vi "Tosca-2P-Frame Rate Counter.vi"(0 "TwoP":T1, 7 "2P Control":refnum<notifier>) -> (15 "error out":errorcluster)   [LabVIEW 2020]
uses:
  Tosca-2P Config.ctl
  <vilib>/DAQmx/read.llb/DAQmx Read (Counter 1D DBL 1Chan NSamp).vi
  <vilib>/Analysis/baseanly.llb/Mean (DBL).vi
  <vilib>/DAQmx/create/channels.llb/DAQmx Create Channel (CI-Period).vi
  <vilib>/DAQmx/configure/timing.llb/DAQmx Timing (Implicit).vi
  <vilib>/DAQmx/miscellaneous.llb/DAQmx Fill In Error Info.vi
  Tosca-2P-Globals.vi
  <vilib>/Analysis/NI_AALBase.lvlib
  <resource>/objmgr/daqmx.rc
panel:
  out "Frame rate (Hz)":dbl
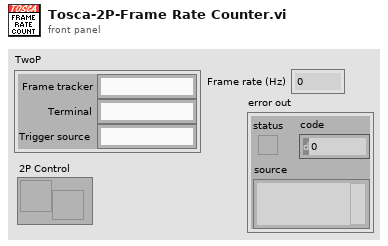
[diagram p1: front panel]
types:
  T1 = typedef "Tosca-2P Config.ctl" = cluster{"Frame tracker":string, "Terminal":string, "Trigger source":string}
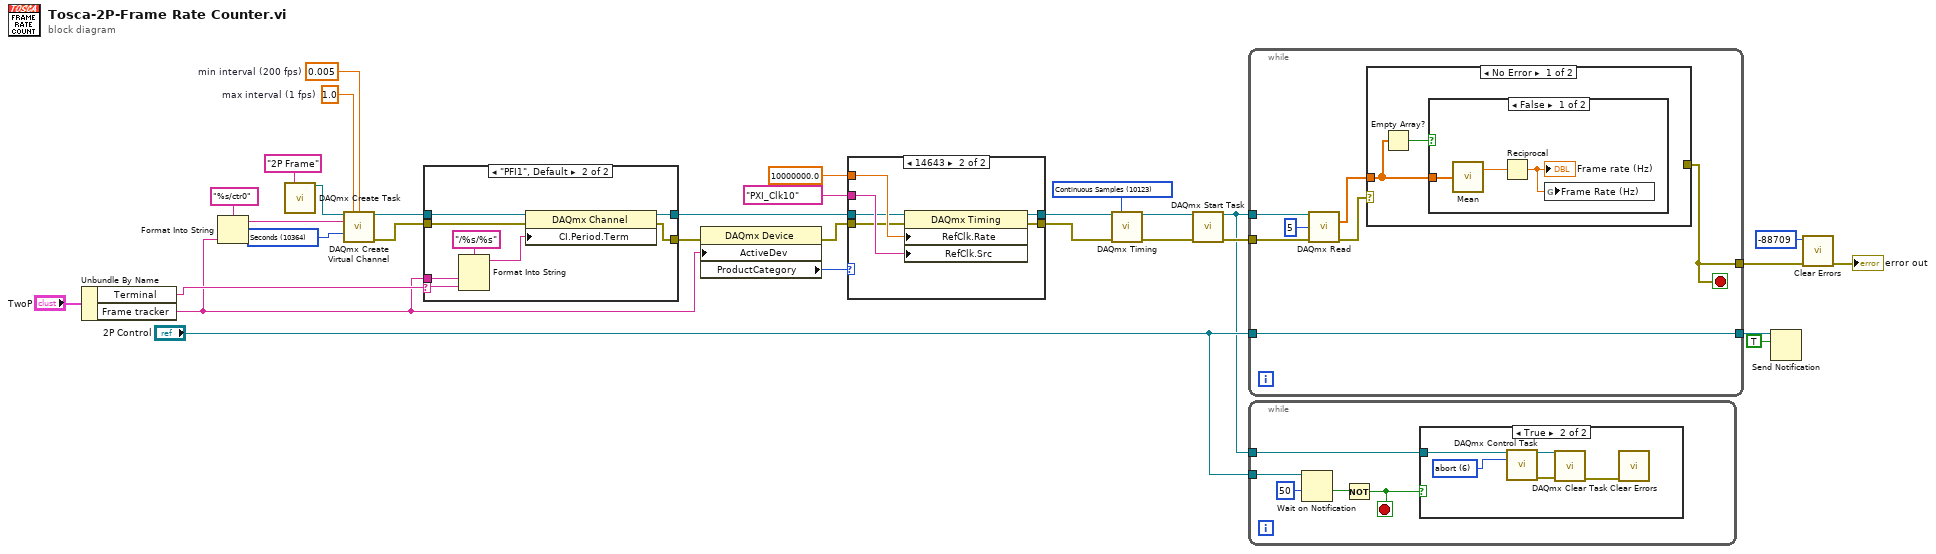
[diagram p0: block diagram]
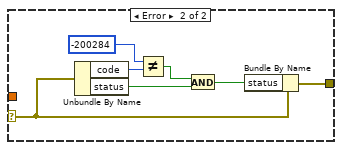
[diagram p6: hidden frame]
diagram:
  w26 = 10364 items=["Seconds"=10364, "Ticks"=10304, "From Custom Scale"=10065] ("units")
  w27 = 0.005  # min interval (200 fps)
  w23 = 1.0  # max interval (1 fps)
  w31 = 10123 items=["Finite Samples"=10178, "Continuous Samples"=10123, "Hardware Timed Single Point"=12522] ("Sample Mode")
  n1 = Unbundle By Name("TwoP") -> ("Terminal"=w2:string, "Frame tracker"=w1:string)
  n2 = Format Into String(format string="%s/ctr0", w1) -> (resulting string=w24:string)  [unwired: 2 in, 1 out]
  n3 = call <vilib>:"DAQmx Create Task.vi"("new task name"="2P Frame") -> ("task out"=w15:refnum<k21>)  [unwired: 13 in, 1 out]
  n4 = call-poly <vilib>:"DAQmx Create Virtual Channel.vi"("task in"=w15, "maximum value"=w23, "minimum value"=w27, "counter"=w24, "units"=w26) -> ("task out"=w7:refnum<k21>, "error out"=w5:errorcluster)  [unwired: 9 in]
  n5 = case shown="\"PFI1\", Default" w2 {
    selector: w2 -> [_ w35]
    tunnel: w7 -> [w33 w39]
    tunnel: [w33 w38] -> w6
    tunnel: w5 -> [w32 w37]
    tunnel: [w32 w36] -> w4
    tunnel: w1 -> [_ w34]
    frame "", "Default" {
    }
    frame "PFI1", Default {
      n6 = Format Into String(format string="/%s/%s", w34, w35) -> (resulting string=w40:string)  [unwired: 2 in, 1 out]
      n7 = property class="DAQmx Channel"(reference=w39, error in=w37, "CI.Period.Term"=w40) -> (reference out=w38:refnum<k21>, error out=w36:errorcluster)
    }
  }
  n8 = property class="DAQmx Device"(error in=w4, "ActiveDev"=w1) -> (error out=w8:errorcluster, "ProductCategory"=w9:i32)  [unwired: 1 in, 1 out]
  n9 = case shown="14643" w9 {
    tunnel: [w43 w49] -> w13
    tunnel: [w42 w48] -> w12
    tunnel: 10000000.0 -> [_ w47]
    tunnel: tag "PXI_Clk10" ("RefClk.Src") -> [_ w46]
    tunnel: w6 -> [w43 w45]
    tunnel: w8 -> [w42 w44]
    frame 0, Default {
    }
    frame 14643 {
      n10 = property class="DAQmx Timing"(reference=w45, error in=w44, "RefClk.Rate"=w47, "RefClk.Src"=w46) -> (reference out=w49:refnum<k21>, error out=w48:errorcluster)
    }
  }
  n11 = call-poly <vilib>:"DAQmx Timing.vi"("task/channels in"=w13, "sample mode"=w31, "error in"=w12) -> ("task out"=w29:refnum<k21>, "error out"=w28:errorcluster)  [unwired: 11 in]
  n12 = call <vilib>:"DAQmx Start Task.vi"("task/channels in"=w29, "error in"=w28) -> ("task out"=w19:refnum<k21>, "error out"=w30:errorcluster)  [unwired: 12 in]
  n13 = while {
    tunnel: w19 -> [w56]
    tunnel: w30 -> [w55]
    tunnel: [w52] -> w17
    tunnel: "2P Control" -> [w50]
    tunnel: [w50] -> w22
    stop <- w52 stop-if-true
    n14 = call-poly <vilib>:"DAQmx Read.vi"("task/channels in"=w56, "number of samples per channel"=5, "error in"=w55) -> ("data"=w54:dbl[], "error out"=w53:errorcluster)  [unwired: 10 in, 1 out]
    n15 = case shown="No Error" w53 {
      selector: w53 -> [_ w64]
      tunnel: w54 -> [w58 _]
      tunnel: [_ w62] -> w52
      frame No Error {
        n16 = Empty Array?(array=w58) -> (empty?=w57:bool)
        n17 = case shown="False" w57 {
          tunnel: w58 -> [w61 _]
          frame False {
            n18 = call-poly <vilib>:"Mean.vi"("X"=w61) -> ("mean"=w60:dbl)  [unwired: 1 out]
            n19 = Reciprocal(x=w60) -> (1/x=w59:dbl)
            "Frame rate (Hz)" <- w59
            n20 = global write "Tosca-2P-Globals.vi" "Frame Rate (Hz)"(w59) -> ()
          }
          frame True {
          }
        }
      }
      frame Error {
        n21 = Unbundle By Name(w64) -> ("code"=w68:i32, "status"=w65:bool)
        n22 = Not Equal?(x=-200284, y=w68) -> (x != y?=w66:bool)
        n23 = And(x=w66, y=w65) -> (x .and. y?=w63:bool)
        n24 = Bundle By Name(cluster=w64, "status"=w63) -> (w62:errorcluster)
      }
    }
  }
  n25 = while {
    tunnel: "2P Control" -> [w71]
    tunnel: w19 -> [w69]
    stop <- w70 stop-if-true
    n26 = Wait on Notification(notifier=w71, timeout in ms (-1)=50) -> (timed out?=w73:bool)  [unwired: 2 in, 3 out]
    n27 = Not(x=w73) -> (.not. x?=w70:bool)
    n28 = case shown="True" w70 {
      tunnel: w69 -> [_ w78]
      frame False {
      }
      frame True {
        w77 = 6 items=["verify"=2, "reserve"=4, "commit"=3, "unreserve"=5, "abort"=6] ("action")
        n29 = call <vilib>:"DAQmx Control Task.vi"("task/channels in"=w78, "action"=w77) -> ("task out"=w76:refnum<k21>, "error out"=w75:errorcluster)  [unwired: 12 in]
        n30 = call <vilib>:"DAQmx Clear Task.vi"("task in"=w76, "error in"=w75) -> ("error out"=w74:errorcluster)  [unwired: 13 in]
        n31 = call <vilib>:"Clear Errors.vi"("error in (no error)"=w74) -> ()  [unwired: 5 in, 2 out]
      }
    }
  }
  n32 = Send Notification(notification=TRUE, notifier=w22) -> ()  [unwired: 1 in, 2 out]
  n33 = call <vilib>:"Clear Errors.vi"("error in (no error)"=w17, "specific error code to clear (0: all)"=-88709) -> ("error out"=→"error out":errorcluster)  [unwired: 4 in, 1 out]
